vi "DSF.Engine.Transfer Group.Errors.vi"   [LabVIEW 2017, in "DSF.Engine.lvlib" / "DSF.Engine.Transfer Group.lvclass"]
uses:
  DSF.Engine.Transfer Group.lvclass
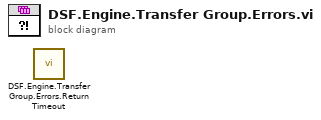
[diagram p0: block diagram]
diagram:
  n1 = call "DSF.Engine.Transfer Group.Errors.Return Timeout.vi"() -> ()  [unwired: 10 in, 2 out]
